vi "Close.vi"(8 "error in (no error)":errorcluster, 11 "NetworkStreamReader in":refnum<class "NetworkStreamReader.lvclass">) -> (0 "error out":errorcluster, 3 "NetworkStreamReader out":refnum<class "NetworkStreamReader.lvclass">)   [LabVIEW 2011, in "NetworkStreamReader.lvclass"]
doc: "This VI closes references internal to the NetworkStreamReader object. This allows memory to be cleaned up effectively."
uses:
  NetworkStreamReader.lvclass
  NetworkStreamReader.lvclass/NetworkStreamReader.ctl
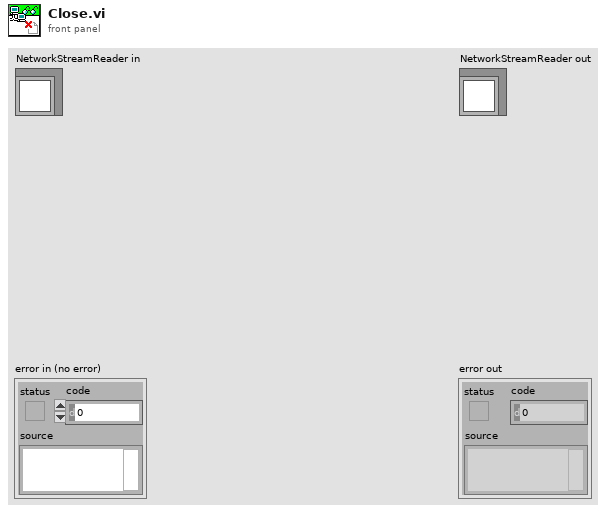
[diagram p1: front panel]
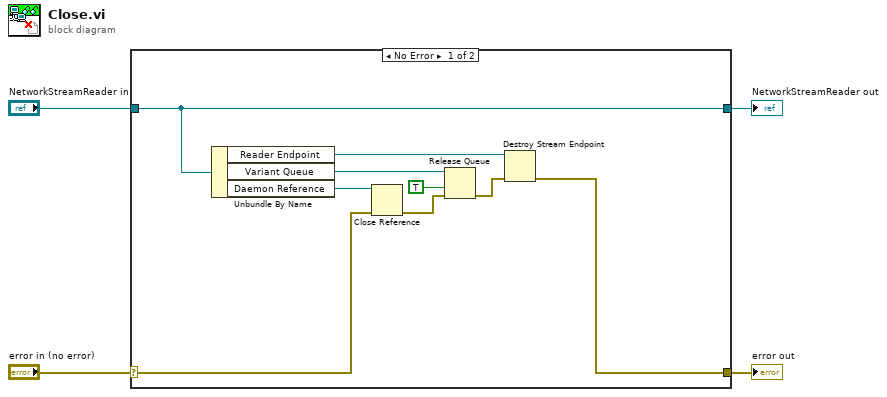
[diagram p0: block diagram]
diagram:
  n1 = case shown="No Error" "error in (no error)" {
    selector: "error in (no error)" -> [w11 w15]
    tunnel: [w6 w15] -> w3
    tunnel: [w13 w14] -> w1
    tunnel: "NetworkStreamReader in" -> [w13 w14]
    frame No Error {
      n2 = Unbundle By Name(w13) -> ("Reader Endpoint"=w8:refnum<k21>, "Variant Queue"=w10:refnum<queue>, "Daemon Reference"=w12:refnum<vi>)
      n3 = Close Reference(reference=w12, error in (no error)=w11) -> (error out=w9:errorcluster)
      n4 = Release Queue(queue=w10, force destroy? (F)=TRUE, error in (no error)=w9) -> (error out=w7:errorcluster)  [unwired: 2 out]
      n5 = Destroy Stream Endpoint(8:w7, 11:w8) -> (0:w6:errorcluster)
    }
    frame Error {
    }
  }
  "error out" <- w3
  "NetworkStreamReader out" <- w1
